vi "FunctionGlobeVar.vi"(6 "Cmd":enum16{"Write", "Read"}(ring), 10 "DataI":cluster{"Data1":i32, "Data2":i32[]}) -> (2 "DataO":cluster{"Data1":i32, "Data2":i32[]})   [LabVIEW 2020]
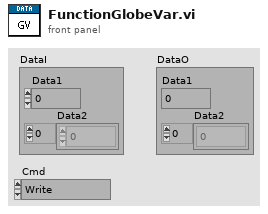
[diagram p1: front panel]
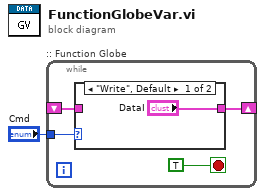
[diagram p0: block diagram]
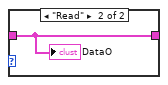
[diagram p2: hidden frame]
diagram:
  n1 = while ":: Function Globe" {
    tunnel: "Cmd" -> [w4]
    shift-right: [w3] -> _
    shift-left: _ -> [w2]
    stop <- TRUE stop-if-true
    n2 = case shown="\"Write\", Default" w4 {
      tunnel: ["DataI" w7] -> w3
      tunnel: w2 -> [_ w7]
      frame "Write", Default {
      }
      frame "Read" {
        "DataO" <- w7
      }
    }
  }
